vi "Content Rect Bounds Separator.vi"(8 "error in (no error)":errorcluster, 10 "Boolean":bool, 11 "DgtlTb in":refnum<class "DigitalTable.lvclass">) -> (0 "error out":errorcluster, 3 "DgtlTb out":refnum<class "DigitalTable.lvclass">)   [LabVIEW 2015, in "DigitalTable.lvclass"]
uses:
  DigitalTable.lvclass
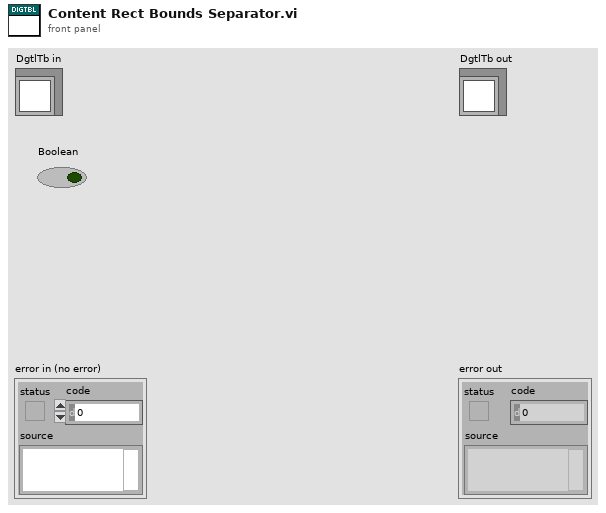
[diagram p1: front panel]
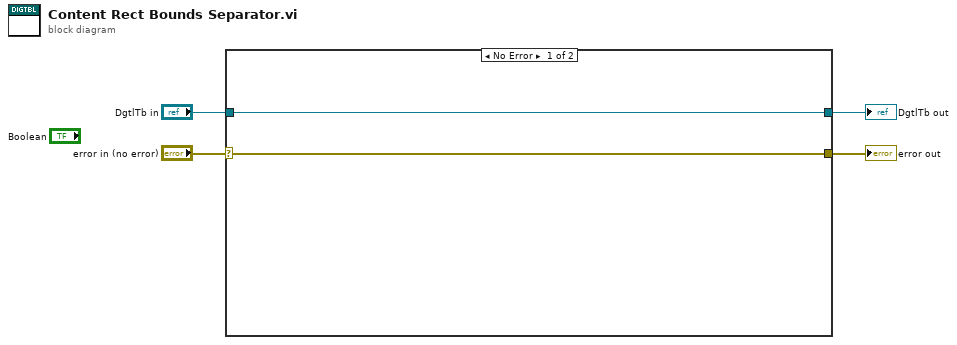
[diagram p0: block diagram]
diagram:
  n1 = case shown="No Error" "error in (no error)" {
    selector: "error in (no error)" -> [w5 w8]
    tunnel: [w5 w8] -> w3
    tunnel: [w6 w7] -> w1
    tunnel: "DgtlTb in" -> [w6 w7]
    frame No Error {
    }
    frame Error {
    }
  }
  "error out" <- w3
  "DgtlTb out" <- w1
